vi "25-09-2020.vi"() -> ()   [LabVIEW 2020]
panel:
  out "Numeric":i32
  in  "Numeric 3":dbl
  out "result":dbl
  in  "Numeric 2":dbl
  in  "Numeric 1":dbl
  in  "Add or Subtract":bool
  out "String":string
  in  "Boolean":bool
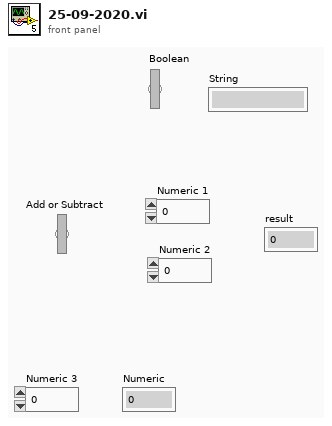
[diagram p1: front panel]
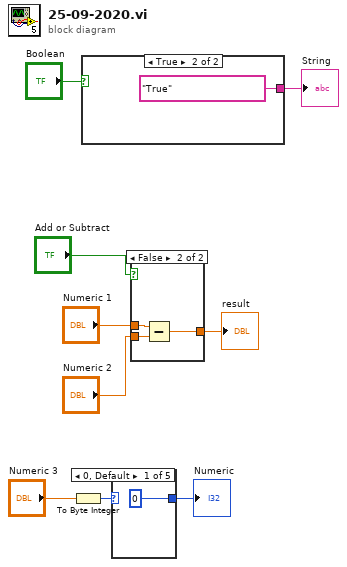
[diagram p0: block diagram]
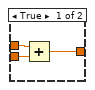
[diagram p6: hidden frame]
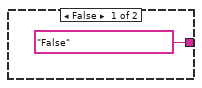
[diagram p7: hidden frame]
diagram:
  n1 = To Byte Integer(number="Numeric 3") -> (8bit integer=w2:i8)
  n2 = case shown="True" "Boolean" {
    tunnel: ["False" "True"] -> w8
    frame False {
    }
    frame True {
    }
  }
  "String" <- w8
  n3 = case shown="0, Default" w2 {
    selector: w2 -> [_ w13 w14 w15 w16]
    tunnel: [0 w13 w14 w15 w16] -> w1
    frame 0, Default {
    }
    frame 1 {
    }
    frame 2 {
    }
    frame 3 {
    }
    frame 4 {
    }
  }
  "Numeric" <- w1
  n4 = case shown="False" "Add or Subtract" {
    tunnel: "Numeric 1" -> [w19 w22]
    tunnel: "Numeric 2" -> [w18 w21]
    tunnel: [w17 w20] -> w4
    frame True {
      n5 = Add(x=w19, y=w18) -> (x+y=w17:dbl)
    }
    frame False {
      n6 = Subtract(x=w22, y=w21) -> (x-y=w20:dbl)
    }
  }
  "result" <- w4
